vi "my Read Controls on Tab from Config File.vi"(4 "error in":errorcluster, 6 "Page Refnum":refnum<vi>, 7 "configuration file path":path) -> (0 "error out":errorcluster, 3 "configuration file path out":path)   [LabVIEW 2019]
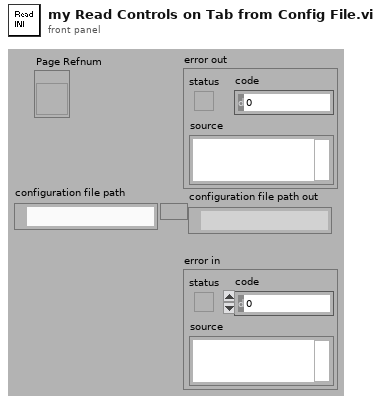
[diagram p1: front panel]
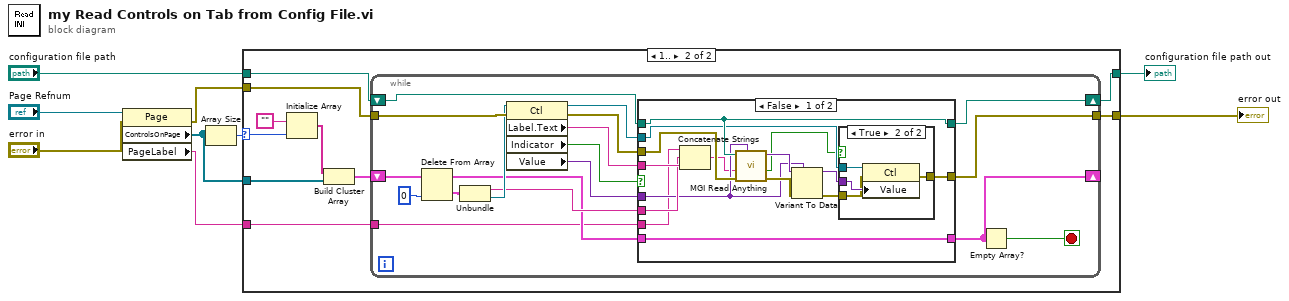
[diagram p0: block diagram]
diagram:
  n1 = property class="Page"(reference="Page Refnum", error in="error in") -> (error out=w7:errorcluster, "ControlsOnPage"=w5:refnum<vi>[], "PageLabel"=w4:string)  [unwired: 1 out]
  n2 = Array Size(array=w5) -> (size(s)=w3:i32)
  n3 = case shown="1.." w3 {
    selector: w3 -> [_ w12]
    tunnel: "configuration file path" -> [w11 w21]
    tunnel: w7 -> [w10 w20]
    tunnel: [w11 w19] -> w1
    tunnel: [w10 w18] -> w6
    tunnel: w5 -> [_ w17]
    tunnel: w4 -> [_ w13]
    frame 0, Default {
    }
    frame 1.. {
      n4 = Initialize Array("", w12) -> (w14:string[])
      n5 = Build Cluster Array(w14, w17) -> (w15:cluster{string, refnum<vi>}[])
      n6 = while {
        shift-right: [w38] -> w19
        shift-left: w21 -> [w39]
        tunnel: w20 -> [w37]
        tunnel: [w35] -> w18
        shift-right: [w25] -> _
        shift-left: w15 -> [w33]
        tunnel: w13 -> [w24]
        stop <- w29 stop-if-true
        n7 = Delete From Array(array=w33, index=0) -> (deleted portion=w32:cluster{string, refnum<vi>}, array with subset deleted=w26:cluster{string, refnum<vi>}[])  [unwired: 1 in]
        n8 = Unbundle(w32) -> (w27:string, w31:refnum<vi>)
        n9 = property class="Ctl"(reference=w31, error in=w37) -> (reference out=w34:refnum<vi>, error out=w36:errorcluster, "Label.Text"=w28:string, "Indicator"=w23:bool, "Value"=w22:variant)
        n10 = case shown="False" w23 {
          tunnel: w39 -> [w50 w61]
          tunnel: [w50 w61] -> w38
          tunnel: w36 -> [w45 w60]
          tunnel: [w44 w60] -> w35
          tunnel: w34 -> [w48 _]
          tunnel: w28 -> [w54 _]
          tunnel: w27 -> [w53 _]
          tunnel: w26 -> [w49 w62]
          tunnel: [w49 w62] -> w25
          tunnel: w24 -> [w41 _]
          tunnel: w22 -> [w42 _]
          frame False {
            n11 = Concatenate Strings(w41, w53, w54) -> (w40:string)
            n12 = call <userlib>:"MGI Read Anything.vi"("Type of Anything"=w42, "Error In"=w45, "Section Name (Name of \"Type of Anything\")"=w40, "Path (dialog)"=w50) -> ("Error Out"=w52:errorcluster, "Found?"=w46:bool, "Anything"=w51:variant)  [unwired: 4 in, 1 out]
            n13 = Variant To Data(error in=w52, type=w42, Variant=w51) -> (data=w47:variant, error out=w43:errorcluster)
            n14 = case shown="True" w46 {
              tunnel: w48 -> [_ w59]
              tunnel: w47 -> [_ w58]
              tunnel: [w55 w57] -> w44
              tunnel: w43 -> [w55 w56]
              frame False {
              }
              frame True {
                n15 = property class="Ctl"(reference=w59, error in=w56, "Value"=w58) -> (error out=w57:errorcluster)  [unwired: 1 out]
              }
            }
          }
          frame True {
          }
        }
        n16 = Empty Array?(array=w25) -> (empty?=w29:bool)
      }
    }
  }
  "error out" <- w6
  "configuration file path out" <- w1
